vi "MissionLocation.vi"(8 "Error In":errorcluster, 11 "PassBouy.lvclass in":refnum<class "PassBouy.lvclass">) -> (0 "Error Out":errorcluster, 2 "element":T1 {"North" format="%#_10f"; "East" format="%#_8f"}, 3 "PassBouy.lvclass out":refnum<class "PassBouy.lvclass">)   [LabVIEW 2012, in "PassBouy.lvclass"]
uses:
  PassBouy.lvclass
  Data/TypeDefs/UTM Location.ctl
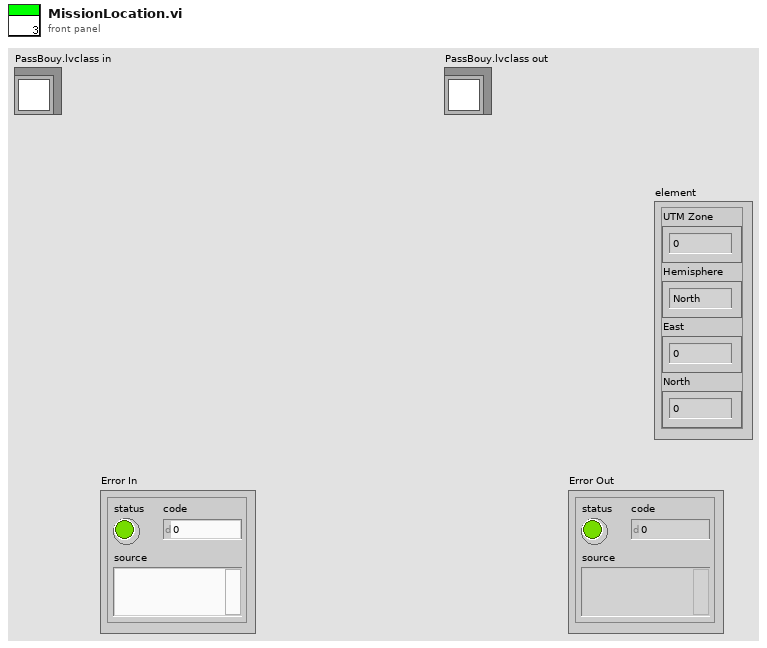
[diagram p1: front panel]
types:
  T1 = typedef "UTM Location.ctl" = cluster{"UTM Zone":dbl, "Hemisphere":enum16{"North", "South"}, "East":dbl, "North":dbl}
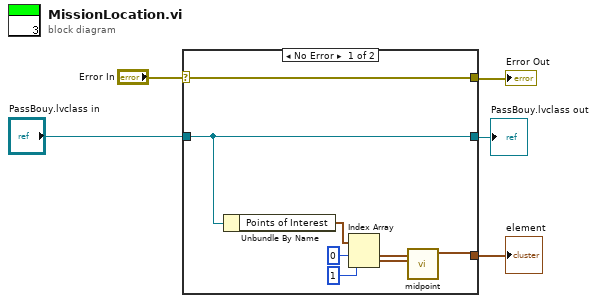
[diagram p0: block diagram]
diagram:
  n1 = case shown="No Error" "Error In" {
    selector: "Error In" -> [w13 w14]
    tunnel: [w13 w14] -> w4
    tunnel: "PassBouy.lvclass in" -> [w12 w15]
    tunnel: [w12 w15] -> w1
    tunnel: [w6 _] -> w3
    frame No Error {
      n2 = Unbundle By Name(w12) -> ("Points of Interest"=w11:T1[])
      n3 = Index Array(array=w11, index #1=0 ("index"), index #2=1 ("index")) -> (element #1=w8:T1, element #2=w7:T1)
      n4 = call "midpoint.vi"("UTM Location 2"=w7, "UTM Location"=w8) -> ("UTM Location 3"=w6:T1)  [unwired: 8 in, 1 out]
    }
    frame Error {
    }
  }
  "Error Out" <- w4
  "element" <- w3
  "PassBouy.lvclass out" <- w1
